vi "Two Color Get Image Type.vi"() -> (4 "Canceled?":bool, 15 "Spooler Code":u8)   [LabVIEW 2016]
uses:
  <vilib>/Utility/miscctls.llb/LVPointTypeDef.ctl
panel:
  in  "Cancel Button":bool
  in  "Salvaged Flour":bool
  in  "Two Color":bool
  # "Select Image Type"
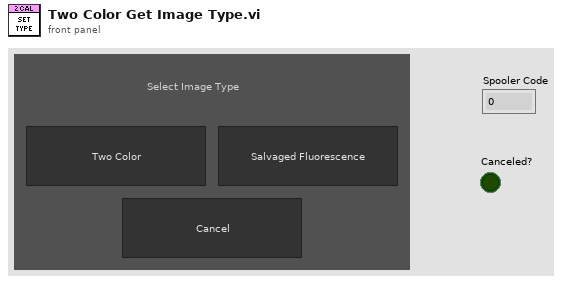
[diagram p1: front panel]
types:
  T1 = enum16{"Always On", "Always Off", "Off While Running"}
  T2 = typedef "LVPointTypeDef.ctl" = cluster{"Horizontal":i16, "Vertical":i16}
  T3 = typedef "LVRectTypeDef.ctl" = cluster{"Left":i16, "Top":i16, "Right":i16, "Bottom":i16}
  T4 = typedef "LVBoundsTypeDef.ctl" = cluster{"Width":u32, "Height":u32}
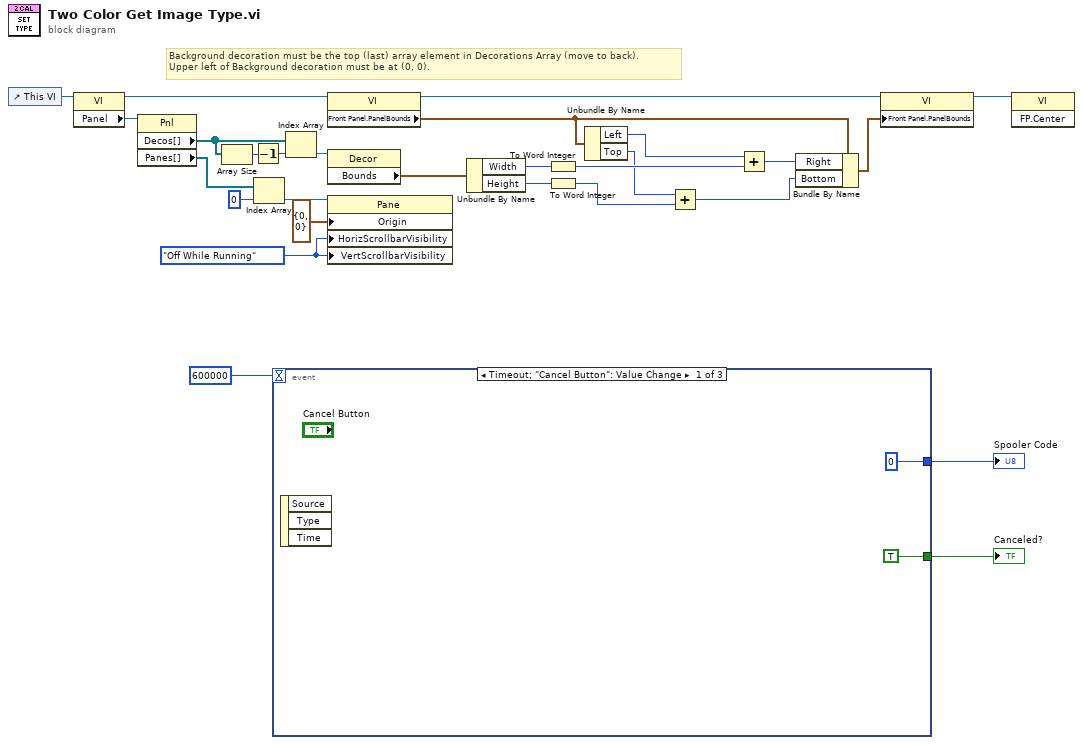
[diagram p0: block diagram]
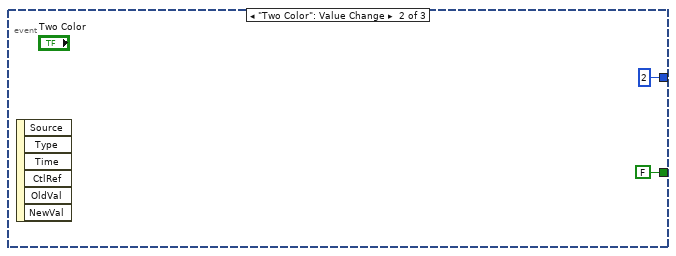
[diagram p2: hidden frame]
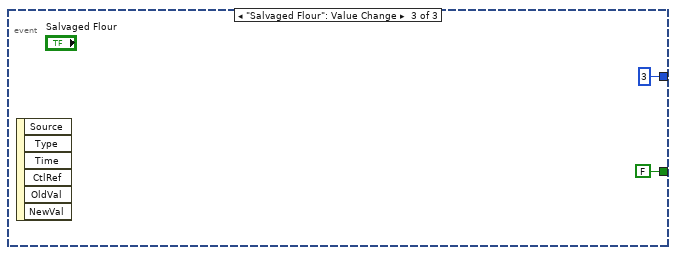
[diagram p3: hidden frame]
diagram:
  w18 = T1."Off While Running" ("Vertical Scrollbar Visibility")
  # "Background decoration must be the top (last) array element in Decorations Array (move to back).\nUpper left of Background decoration must be at (0, 0)."
  n1 = control-ref of="This VI"() -> (w11:refnum<vi>)
  n2 = property class="VI"(reference=w11) -> (reference out=w19:refnum<vi>, "Panel"=w12:refnum<vi>)  [unwired: 1 in, 1 out]
  n3 = property class="Pnl"(reference=w12) -> ("Decos[]"=w10:refnum<vi>[], "Panes[]"=w15:refnum<vi>[])  [unwired: 1 in, 2 out]
  n4 = Array Size(array=w10) -> (size(s)=w8:i32)
  n5 = Decrement(x=w8) -> (x-1=w9:i32)
  n6 = Index Array(array=w15, index=0) -> (element=w14:refnum<vi>)
  n7 = event shown="[0] Timeout;  \"Cancel Button\": Value Change" {
    selector: _ -> [_ _ _]
    dyn-events: _ -> [_ _ _]
    timeout: 600000 -> [_ _ _]
    tunnel: [u8 0 u8 2 u8 3] -> w2
    tunnel: [TRUE FALSE FALSE] -> w1
    event Timeout; "Cancel Button": Value Change {
      n8 = event-data() -> ()  [unwired: 1 in, 3 out]
    }
    event "Two Color": Value Change {
      n9 = event-data() -> ()  [unwired: 1 in, 6 out]
    }
    event "Salvaged Flour": Value Change {
      n10 = event-data() -> ()  [unwired: 1 in, 6 out]
    }
  }
  "Spooler Code" <- w2
  "Canceled?" <- w1
  n11 = Index Array(array=w10, index=w9) -> (element=w17:refnum<vi>)
  n12 = property class="VI"(reference=w19) -> (reference out=w21:refnum<vi>, "Front Panel.PanelBounds"=w22:T3)  [unwired: 1 in, 1 out]
  n13 = property class="Decor"(reference=w17) -> ("Bounds"=w20:T4)  [unwired: 1 in, 2 out]
  n14 = property class="Pane"(reference=w14, "Origin"=T2 {"Horizontal"=0, "Vertical"=0}, "HorizScrollbarVisibility"=w18, "VertScrollbarVisibility"=w18) -> ()  [unwired: 1 in, 2 out]
  n15 = Unbundle By Name(w20) -> ("Width"=w25:u32, "Height"=w28:u32)
  n16 = To Word Integer(number=w25) -> (16bit integer=w27:i16)
  n17 = To Word Integer(number=w28) -> (16bit integer=w6:i16)
  n18 = Unbundle By Name(w22) -> ("Left"=w24:i16, "Top"=w7:i16)
  n19 = Add(x=w7, y=w6) -> (x+y=w5:i16)
  n20 = Add(x=w24, y=w27) -> (x+y=w26:i16)
  n21 = Bundle By Name(cluster=w22, "Right"=w26, "Bottom"=w5) -> (w23:T3)
  n22 = property class="VI"(reference=w21, "Front Panel.PanelBounds"=w23) -> (reference out=w4:refnum<vi>)  [unwired: 1 in, 1 out]
  n23 = invoke class="VI" method="FP.Center"(reference=w4) -> ()  [unwired: 2 in, 3 out]
